vi "Read control functions.vi"(8 "error in":errorcluster, 11 "user tag bus module configuration In":refnum<class "TEST CONFIGURATION.lvclass">) -> (0 "error out":errorcluster, 2 "control functions":T1[](array[typedef]) {"output range"."output low" format="%.2f"; "output range"."output high" format="%.2f"}, 3 "user tag bus module configuration Out":refnum<class "TEST CONFIGURATION.lvclass">)   [LabVIEW 2013, in "configuration tests.lvlib" / "TEST CONFIGURATION.lvclass"]
uses:
  TEST CONFIGURATION.lvclass
  control module configuration.ctl
  <vilib>/NI/Tag Bus Module Framework/channel/TBM channel.lvclass
  gains.ctl
  TEST CONFIGURATION.lvclass/TEST CONFIGURATION.ctl
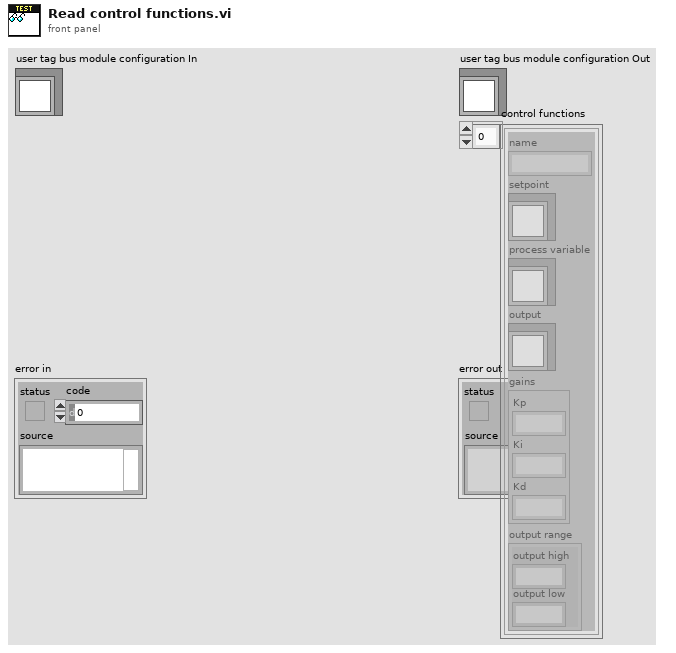
[diagram p1: front panel]
types:
  T1 = typedef "configuration tests.lvlib/TEST CONFIGURATION.lvclass/control module configuration.ctl" = cluster{"name":string, "setpoint":refnum<class "TBM channel.lvclass">, "process variable":refnum<class "TBM channel.lvclass">, "output":refnum<class "TBM channel.lvclass">, "gains":T2, "output range":cluster{"output high":dbl, "output low":dbl}}
  T2 = typedef "configuration tests.lvlib/TEST CONFIGURATION.lvclass/gains.ctl" = cluster{"Kp":dbl, "Ki":dbl, "Kd":dbl}
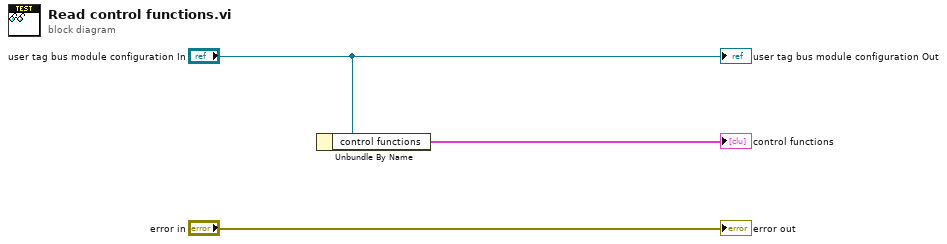
[diagram p0: block diagram]
diagram:
  n1 = Unbundle By Name("user tag bus module configuration In") -> ("control functions"=→"control functions":T1[])
  "error out" <- "error in"
  "user tag bus module configuration Out" <- "user tag bus module configuration In"
